vi "Timer.vi"(8 "error in":errorcluster, 10 "TimetoElapsed (s)":dbl, 11 "Todo":T1) -> (0 "error out":errorcluster, 2 "Elapsed ?":bool, 3 "TimeElapsed (s)":dbl format="%#_g s")   [LabVIEW 2020]
doc: "Timer is FGV allow to initialize and give elapsed time from start tick"
uses:
  Controls/Timer_todo.ctl
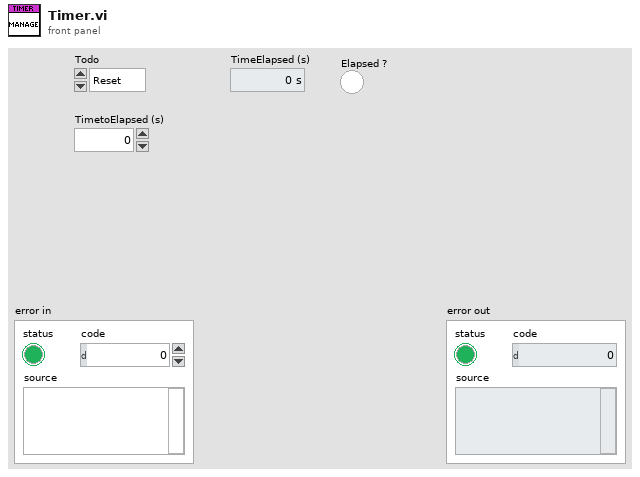
[diagram p1: front panel]
types:
  T1 = typedef "Timer_todo.ctl" = enum16{"Reset", "Elapsed"}
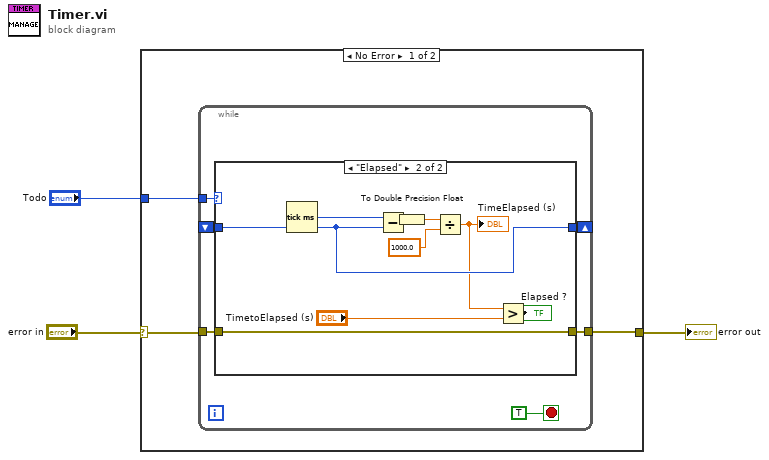
[diagram p0: block diagram]
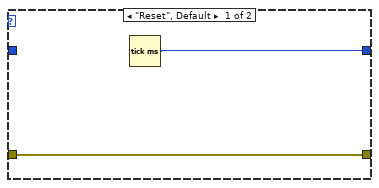
[diagram p2: hidden frame]
diagram:
  n1 = case shown="No Error" "error in" {
    selector: "error in" -> [w6 w24]
    tunnel: [w5 w24] -> w2
    tunnel: "Todo" -> [w4 _]
    frame No Error {
      n2 = while {
        tunnel: w6 -> [w11]
        tunnel: [w10] -> w5
        tunnel: w4 -> [w9]
        shift-right: [w8] -> _
        shift-left: _ -> [w7]
        stop <- TRUE stop-if-true
        n3 = case shown="\"Elapsed\"" w9 {
          tunnel: w11 -> [w14 w23]
          tunnel: [w14 w23] -> w10
          tunnel: [w13 w22] -> w8
          tunnel: w7 -> [_ w22]
          frame "Reset", Default {
            n4 = Tick Count (ms)() -> (millisecond timer value=w13:u32)
          }
          frame "Elapsed" {
            n5 = Tick Count (ms)() -> (millisecond timer value=w21:u32)
            n6 = Subtract(x=w21, y=w22) -> (x-y=w20:u32)
            n7 = To Double Precision Float(number=w20) -> (double precision float=w18:dbl)
            n8 = Divide(x=w18, y=1000.0) -> (x/y=w17:dbl)
            "TimeElapsed (s)" <- w17
            n9 = Greater?(x=w17, y="TimetoElapsed (s)") -> (0:→"Elapsed ?":bool)
          }
        }
      }
    }
    frame Error {
    }
  }
  "error out" <- w2
